vi "RTS Check Time Index.vi"(5 "Station #":u8=1 min=1 max=8 step=1, 6 "Door Output Relays":T4, 7 "Relay #":u8=1 min=1 max=3 step=1, 8 "Error In":errorcluster, 10 "Input":refnum<class "Modbus Master.lvclass">, 11 "Chamber 1-1 Input":T1[](array[typedef]) {"Start Time" format="%<%X\n%x>T"; "End Time" format="%<%X\n%x>T"}) -> (0 "Error Out":errorcluster, 2 "Output":refnum<class "Modbus Master.lvclass">, 3 "Chamber 1-1 Output":T1[](array[typedef]) {"Start Time" format="%<%X\n%x>T"; "End Time" format="%<%X\n%x>T"}, 4 "Index Number":i32)   [LabVIEW 2016]
uses:
  Type Definitions/RTS Door Ops Client.ctl
  Type Definitions/RTS Door Opening Schedule.ctl
  Type Definitions/RTS Door Ops Sequence.ctl
  <vilib>/NI/Modbus Library/API/Master/Modbus Master.lvclass
  Drivers/WAGO 750-881/Type Definitions/Wago Door Relays.ctl
panel:
  # "Chamber Conditions:"
  # "Chamber Conditions:"
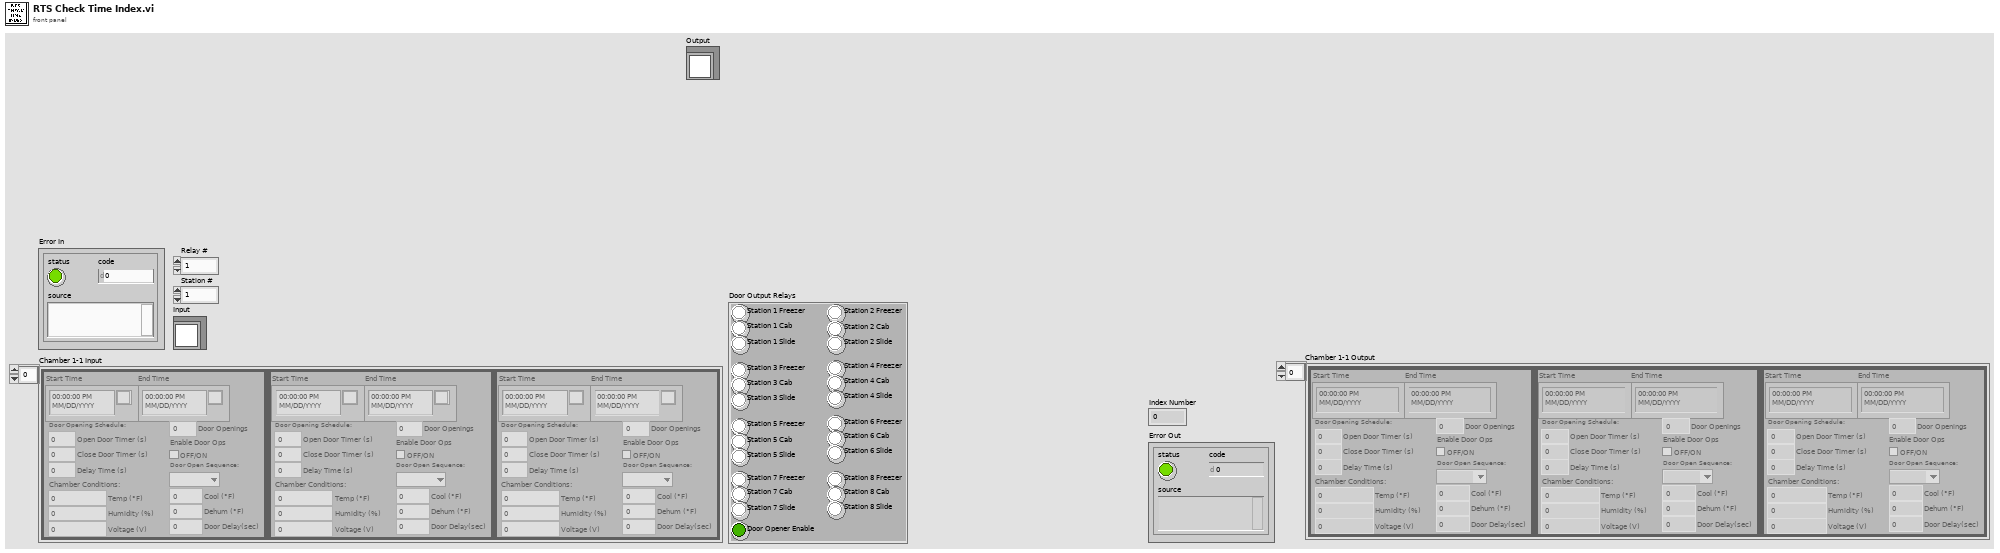
[diagram p1: front panel]
types:
  T1 = typedef "RTS Door Ops Client.ctl" = cluster{"End Time":timestamp, "Start Time":timestamp, "Door Opening Schedule:":T2, "Enable Door Ops":bool, "Door Openings":u32, "Temp (°F)":dbl, "Humidity (%)":dbl, "Voltage (V)":dbl, "Door Open Sequence:":T3, "Door Delay(sec)":dbl, "Dehum (°F)":dbl, "Cool (°F)":dbl}
  T2 = typedef "RTS Door Opening Schedule.ctl" = cluster{"Open Door Timer (s)":dbl, "Delay Time (s)":dbl, "Close Door Timer (s)":dbl}
  T3 = typedef "RTS Door Ops Sequence.ctl" = enum16{"", "1st", "2nd", "3rd"}
  T4 = typedef "Wago Door Relays.ctl" = cluster{"Station 1 Freezer":bool, "Station 1 Cab":bool, "Station 1 Slide":bool, "Station 2 Freezer":bool, "Station 2 Cab":bool, "Station 2 Slide":bool, "Station 3 Freezer":bool, "Station 3 Cab":bool, "Station 3 Slide":bool, "Station 4 Freezer":bool, "Station 4 Cab":bool, "Station 4 Slide":bool, "Station 5 Freezer":bool, "Station 5 Cab":bool, "Station 5 Slide":bool, "Station 6 Freezer":bool, "Station 6 Cab":bool, "Station 6 Slide":bool, "Station 7 Freezer":bool, "Station 7 Cab":bool, "Station 7 Slide":bool, "Station 8 Freezer":bool, "Station 8 Cab":bool, "Station 8 Slide":bool, "Door Opener Enable":bool}
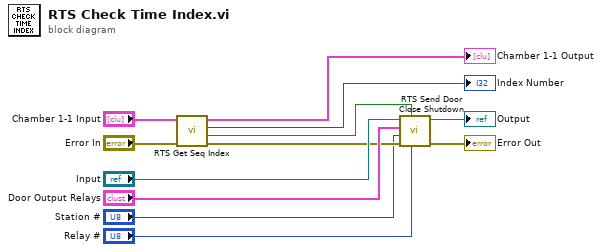
[diagram p0: block diagram]
diagram:
  n1 = call "RTS Get Seq Index.vi"("error in (no error)"="Error In", "Chamber 1-1 Input"="Chamber 1-1 Input") -> ("Error Out"=w6:errorcluster, "Times Up?"=w3:bool, "Index Number"=→"Index Number":i32, "Chamber 1-1 Output"=→"Chamber 1-1 Output":T1[])  [unwired: 6 in]
  n2 = call "RTS Send Door Close Shutdown.vi"("Relay #"="Relay #", "Times Up?"=w3, "Error In"=w6, "Station #"="Station #", "Door Output Relays"="Door Output Relays", "Modbus Master in"="Input") -> ("Error Out"=→"Error Out":errorcluster, "Modbus Master out"=→"Output":refnum<class "Modbus Master.lvclass">)  [unwired: 4 in]
